vi "Squared Driving.vi"(8 "Translation Joystick":dbl format="%#_13g", 9 "Rotation Joystick":dbl format="%#_13g", 10 "Translation Power":dbl=1.0, 11 "Rotation Power":dbl=1.4) -> (2 "Y":dbl, 3 "X":dbl)   [LabVIEW 2018]
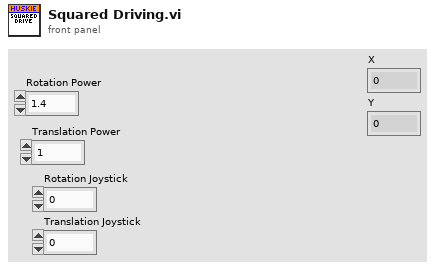
[diagram p1: front panel]
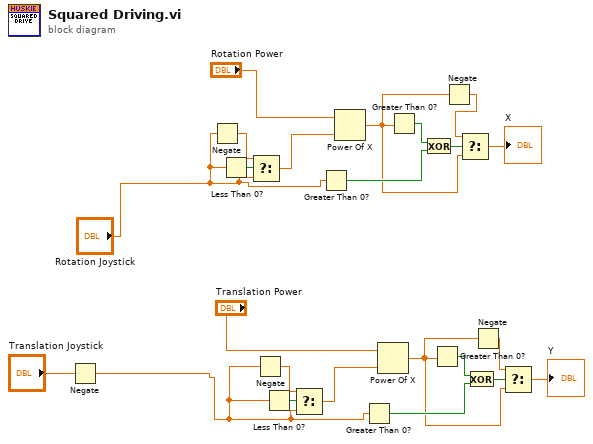
[diagram p0: block diagram]
diagram:
  n1 = Negate(x="Translation Joystick") -> (-x=w3:dbl)
  n2 = Negate(x="Rotation Joystick") -> (-x=w22:dbl)
  n3 = Less Than 0?(x="Rotation Joystick") -> (x < 0?=w20:bool)
  n4 = Select(t=w22, s=w20, f="Rotation Joystick") -> (s? t:f=w21:dbl)
  n5 = Negate(x=w3) -> (-x=w14:dbl)
  n6 = Less Than 0?(x=w3) -> (x < 0?=w12:bool)
  n7 = Select(t=w14, s=w12, f=w3) -> (s? t:f=w13:dbl)
  n8 = Greater Than 0?(x="Rotation Joystick") -> (x > 0?=w18:bool)
  n9 = Power Of X(1:w21, 2:"Rotation Power") -> (0:w15:dbl)
  n10 = Greater Than 0?(x=w3) -> (x > 0?=w10:bool)
  n11 = Power Of X(1:w13, 2:"Translation Power") -> (0:w6:dbl)
  n12 = Greater Than 0?(x=w15) -> (x > 0?=w19:bool)
  n13 = Exclusive Or(1:w18, 2:w19) -> (0:w17:bool)
  n14 = Greater Than 0?(x=w6) -> (x > 0?=w11:bool)
  n15 = Negate(x=w15) -> (-x=w16:dbl)
  n16 = Select(t=w16, s=w17, f=w15) -> (s? t:f=→"X":dbl)
  n17 = Exclusive Or(1:w10, 2:w11) -> (0:w9:bool)
  n18 = Negate(x=w6) -> (-x=w7:dbl)
  n19 = Select(t=w7, s=w9, f=w6) -> (s? t:f=→"Y":dbl)
